vi "3 D Ang Pos for 6 Field-Int.vi"(6 "With Respect To:":enum16{"Referenced", "UnReferenced"}(ring), 7 "LE and RE 2D coils":bool, 8 "Reference index":i32, 9 "3D Convention":T1(ring), 10 "Field Gains":i32[](array[numeric]), 11 "3D Voltage Data":dbl[][](array[numeric]) format="%.2f") -> (3 "3D Position":dbl[][](array[numeric]) format="%.2f")   [LabVIEW 2016]
panel:
  # "Copyright Americo A. Migliaccio (c) 2002 All Rights Reserved by Author"
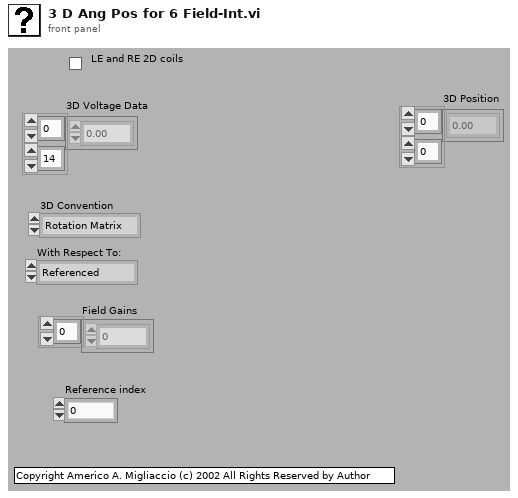
[diagram p1: front panel]
types:
  T1 = enum16{"Rotation Matrix", "Rotation Vectors", "Quaternions", "Fick Angles", "Helmholtz Angles"}
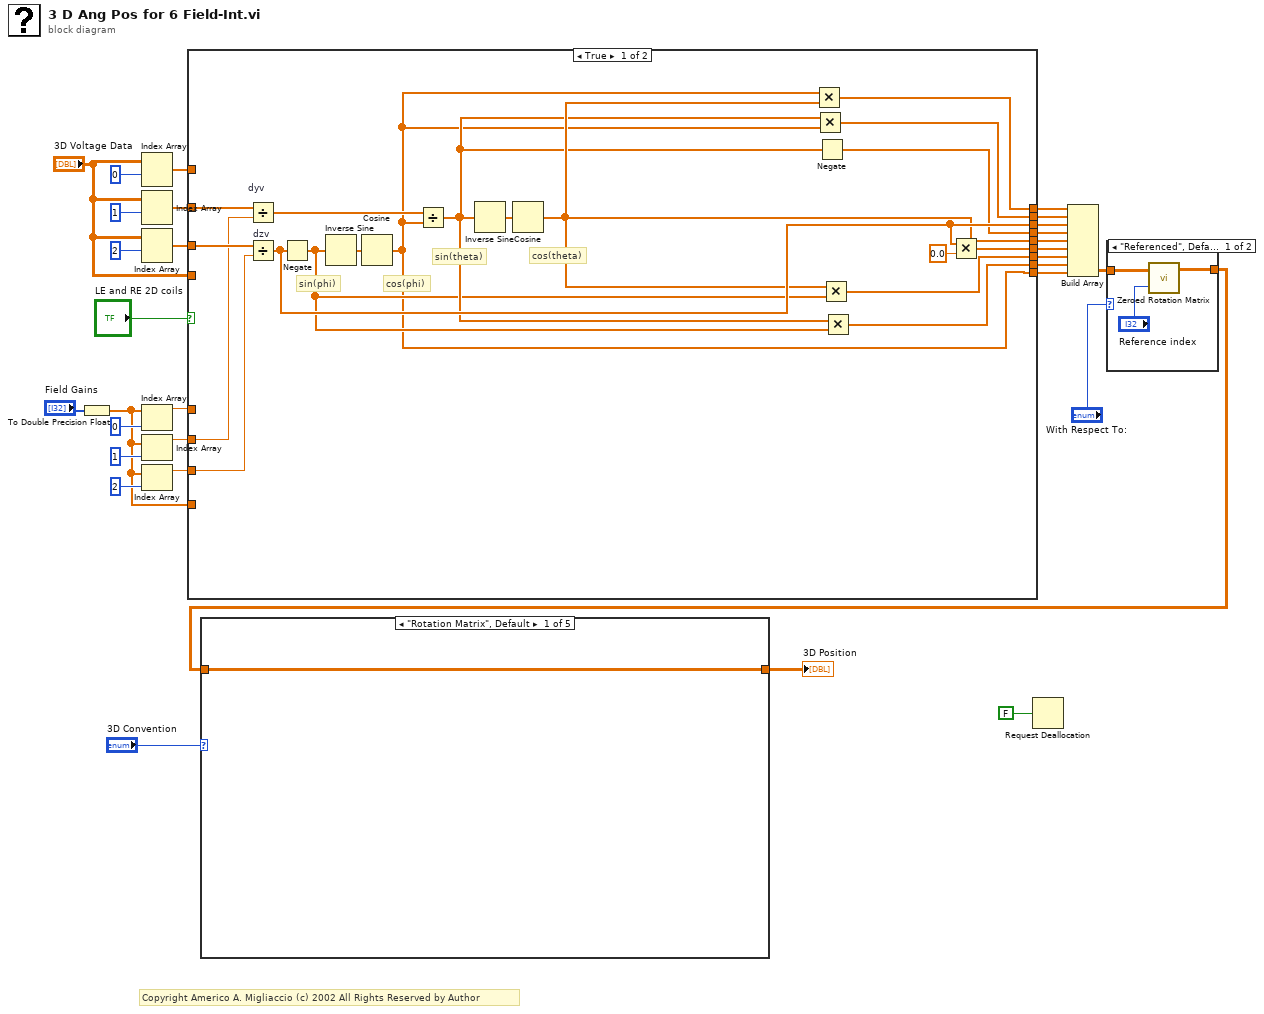
[diagram p0: block diagram]
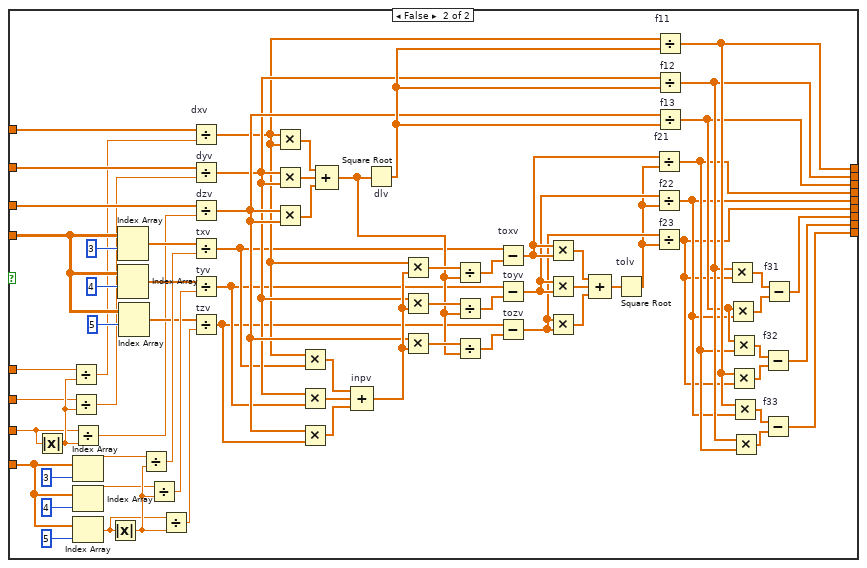
[diagram p2: hidden frame]
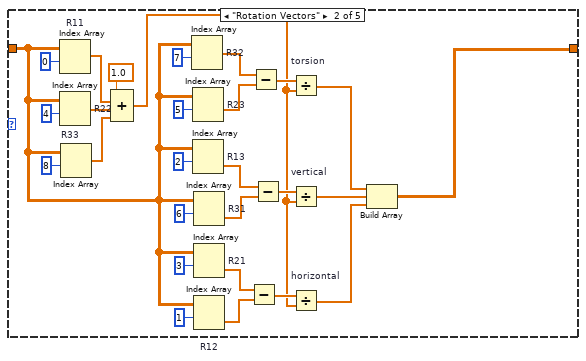
[diagram p4: hidden frame]
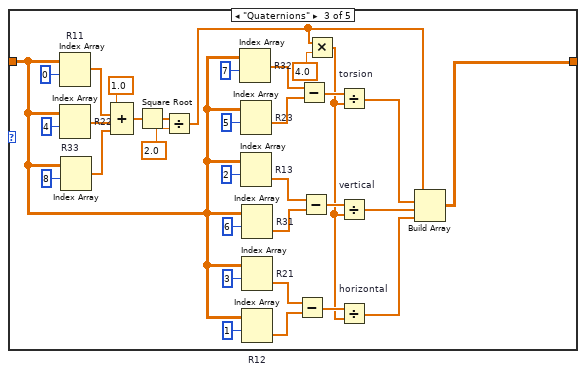
[diagram p5: hidden frame]
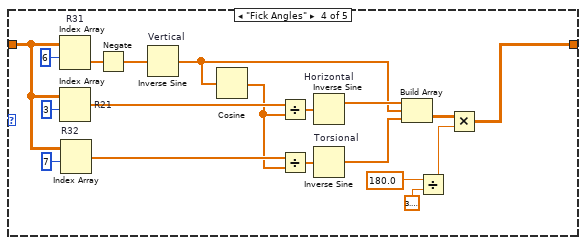
[diagram p6: hidden frame]
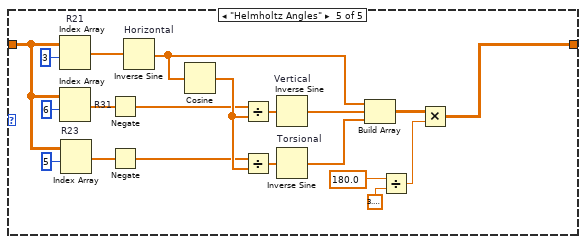
[diagram p7: hidden frame]
diagram:
  # "Copyright Americo A. Migliaccio (c) 2002 All Rights Reserved by Author"
  n1 = To Double Precision Float(number="Field Gains") -> (double precision float=w5:dbl[])
  n2 = Index Array(array="3D Voltage Data", index (row)=0 ("Index (row)")) -> (element=w9:dbl[])  [unwired: 1 in]
  n3 = Index Array(array="3D Voltage Data", index (row)=1 ("Index (row)")) -> (element=w31:dbl[])  [unwired: 1 in]
  n4 = Index Array(array="3D Voltage Data", index (row)=2 ("Index (row)")) -> (element=w30:dbl[])  [unwired: 1 in]
  n5 = Index Array(array=w5, index=0 ("Index")) -> (element=w1:dbl)
  n6 = Index Array(array=w5, index=1 ("Index")) -> (element=w2:dbl)
  n7 = Index Array(array=w5, index=2 ("Index")) -> (element=w3:dbl)
  n8 = case shown="True" "LE and RE 2D coils" {
    tunnel: w31 -> [w50 w122]
    tunnel: w30 -> [w49 w121]
    tunnel: w1 -> [_ w56]
    tunnel: w2 -> [w44 w55]
    tunnel: w3 -> [w43 w54]
    tunnel: [w42 w83] -> w22
    tunnel: [w41 w82] -> w21
    tunnel: [w40 w81] -> w20
    tunnel: [w32 w80] -> w19
    tunnel: [w38 w79] -> w18
    tunnel: [w39 w78] -> w17
    tunnel: [w37 w77] -> w16
    tunnel: [w34 w76] -> w15
    tunnel: [w33 w75] -> w14
    tunnel: w9 -> [_ w74]
    tunnel: "3D Voltage Data" -> [_ w59]
    tunnel: w5 -> [_ w58]
    frame True {
      # "sin(phi)"
      # "cos(phi)"
      # "cos(theta)"
      # "sin(theta)"
      n9 = Divide "dyv"(x=w50, y=w44) -> (x/y=w48:dbl[])
      n10 = Divide "dzv"(x=w49, y=w43) -> (x/y=w40:dbl[])
      n11 = Negate(x=w40) -> (-x=w35:dbl[])
      n12 = Inverse Sine(1:w35) -> (0:w47:dbl[])
      n13 = Cosine(x=w47) -> (cos(x)=w33:dbl[])
      n14 = Divide(x=w48, y=w33) -> (x/y=w36:dbl[])
      n15 = Inverse Sine(1:w36) -> (0:w46:dbl[])
      n16 = Cosine(x=w46) -> (cos(x)=w38:dbl[])
      n17 = Multiply(x=w33, y=w38) -> (x*y=w42:dbl[])
      n18 = Multiply(x=w36, y=w33) -> (x*y=w41:dbl[])
      n19 = Negate(x=w36) -> (-x=w32:dbl[])
      n20 = Multiply(x=w38, y=w35) -> (x*y=w37:dbl[])
      n21 = Multiply(x=w36, y=w35) -> (x*y=w34:dbl[])
      n22 = Multiply(x=w40, y=0.0 ("Index")) -> (x*y=w39:dbl[])
    }
    frame False {
      n23 = Absolute Value(x=w54) -> (abs(x)=w57:dbl)
      n24 = Divide(x=w56, y=w57) -> (x/y=w53:dbl)
      n25 = Divide(x=w55, y=w57) -> (x/y=w52:dbl)
      n26 = Divide(x=w54, y=w57) -> (x/y=w51:dbl)
      n27 = Index Array(array=w58, index=3 ("Index")) -> (element=w117:dbl)
      n28 = Index Array(array=w58, index=4 ("Index")) -> (element=w116:dbl)
      n29 = Index Array(array=w58, index=5 ("Index")) -> (element=w115:dbl)
      n30 = Absolute Value(x=w115) -> (abs(x)=w118:dbl)
      n31 = Index Array(array=w59, index (row)=3 ("Index (row)")) -> (element=w120:dbl[])  [unwired: 1 in]
      n32 = Index Array(array=w59, index (row)=4 ("Index (row)")) -> (element=w119:dbl[])  [unwired: 1 in]
      n33 = Index Array(array=w59, index (row)=5 ("Index (row)")) -> (element=w71:dbl[])  [unwired: 1 in]
      n34 = Divide(x=w117, y=w118) -> (x/y=w114:dbl)
      n35 = Divide(x=w116, y=w118) -> (x/y=w113:dbl)
      n36 = Divide(x=w115, y=w118) -> (x/y=w112:dbl)
      n37 = Divide "dxv"(x=w74, y=w53) -> (x/y=w70:dbl[])
      n38 = Divide "dyv"(x=w122, y=w52) -> (x/y=w72:dbl[])
      n39 = Divide "dzv"(x=w121, y=w51) -> (x/y=w73:dbl[])
      n40 = Divide "txv"(x=w120, y=w114) -> (x/y=w62:dbl[])
      n41 = Divide "tyv"(x=w119, y=w113) -> (x/y=w61:dbl[])
      n42 = Divide "tzv"(x=w71, y=w112) -> (x/y=w60:dbl[])
      n43 = Multiply(x=w70, y=w70) -> (x*y=w105:dbl[])
      n44 = Multiply(x=w72, y=w72) -> (x*y=w104:dbl[])
      n45 = Multiply(x=w73, y=w73) -> (x*y=w103:dbl[])
      n46 = Multiply(x=w70, y=w62) -> (x*y=w102:dbl[])
      n47 = Multiply(x=w72, y=w61) -> (x*y=w101:dbl[])
      n48 = Multiply(x=w73, y=w60) -> (x*y=w100:dbl[])
      n49 = Compound Arithmetic op=ADD ("dlv")(w105, w104, w103) -> (w66:dbl[])
      n50 = Compound Arithmetic op=ADD "inpv"(w102, w101, w100) -> (w99:dbl[])
      n51 = Square Root "dlv"(x=w66) -> (sqrt(x)=w94:dbl[])
      n52 = Multiply(x=w70, y=w99) -> (x*y=w69:dbl[])
      n53 = Multiply(x=w72, y=w99) -> (x*y=w68:dbl[])
      n54 = Multiply(x=w73, y=w99) -> (x*y=w67:dbl[])
      n55 = Divide(x=w69, y=w66) -> (x/y=w65:dbl[])
      n56 = Divide(x=w68, y=w66) -> (x/y=w64:dbl[])
      n57 = Divide(x=w67, y=w66) -> (x/y=w63:dbl[])
      n58 = Subtract "toxv"(x=w62, y=w65) -> (x-y=w93:dbl[])
      n59 = Subtract "toyv"(x=w61, y=w64) -> (x-y=w92:dbl[])
      n60 = Subtract "tozv"(x=w60, y=w63) -> (x-y=w91:dbl[])
      n61 = Multiply(x=w93, y=w93) -> (x*y=w97:dbl[])
      n62 = Multiply(x=w92, y=w92) -> (x*y=w98:dbl[])
      n63 = Multiply(x=w91, y=w91) -> (x*y=w96:dbl[])
      n64 = Compound Arithmetic op=ADD ("dlv")(w97, w98, w96) -> (w95:dbl[])
      n65 = Square Root "tolv"(x=w95) -> (sqrt(x)=w90:dbl[])
      n66 = Divide "f21"(x=w93, y=w90) -> (x/y=w80:dbl[])
      n67 = Divide "f22"(x=w92, y=w90) -> (x/y=w79:dbl[])
      n68 = Divide "f23"(x=w91, y=w90) -> (x/y=w78:dbl[])
      n69 = Divide "f11"(x=w70, y=w94) -> (x/y=w83:dbl[])
      n70 = Divide "f12"(x=w72, y=w94) -> (x/y=w82:dbl[])
      n71 = Divide "f13"(x=w73, y=w94) -> (x/y=w81:dbl[])
      n72 = Multiply(x=w82, y=w78) -> (x*y=w89:dbl[])
      n73 = Multiply(x=w81, y=w79) -> (x*y=w88:dbl[])
      n74 = Multiply(x=w81, y=w80) -> (x*y=w87:dbl[])
      n75 = Multiply(x=w83, y=w78) -> (x*y=w86:dbl[])
      n76 = Multiply(x=w83, y=w79) -> (x*y=w85:dbl[])
      n77 = Multiply(x=w82, y=w80) -> (x*y=w84:dbl[])
      n78 = Subtract "f32"(x=w87, y=w86) -> (x-y=w76:dbl[])
      n79 = Subtract "f33"(x=w85, y=w84) -> (x-y=w75:dbl[])
      n80 = Subtract "f31"(x=w89, y=w88) -> (x-y=w77:dbl[])
    }
  }
  n81 = Request Deallocation(FALSE ("flag")) -> ()
  n82 = Build Array(w22, w21, w20, w19, w18, w17, w16, w15, w14) -> (w13:dbl[][])
  n83 = case shown="\"Referenced\", Default" "With Respect To:" {
    tunnel: w13 -> [w125 w126]
    tunnel: [w123 w126] -> w8
    frame "Referenced", Default {
      n84 = call "Zeroed Rotation Matrix.vi"("Reference index"="Reference index", "Unreferenced Rotation Matrix"=w125) -> ("Referenced Rotation Matrix"=w123:dbl[][])  [unwired: 1 in]
    }
    frame "UnReferenced" {
    }
  }
  n85 = case shown="\"Rotation Matrix\", Default" "3D Convention" {
    tunnel: w8 -> [w127 w142 w175 w204 w224]
    tunnel: [w127 w128 w161 w189 w208] -> w11
    frame "Rotation Matrix", Default {
    }
    frame "Rotation Vectors" {
      n86 = Index Array "R11"(array=w142, index (row)=0 ("Index (row)")) -> (element=w150:dbl[])  [unwired: 1 in]
      n87 = Index Array "R22"(array=w142, index (row)=4 ("Index (row)")) -> (element=w151:dbl[])  [unwired: 1 in]
      n88 = Index Array "R33"(array=w142, index (row)=8 ("Index (row)")) -> (element=w152:dbl[])  [unwired: 1 in]
      n89 = Compound Arithmetic op=ADD(1.0, w150, w151, w152) -> (w132:dbl[])
      n90 = Index Array "R32"(array=w142, index (row)=7 ("Index (row)")) -> (element=w141:dbl[])  [unwired: 1 in]
      n91 = Index Array "R23"(array=w142, index (row)=5 ("Index (row)")) -> (element=w140:dbl[])  [unwired: 1 in]
      n92 = Index Array "R13"(array=w142, index (row)=2 ("Index (row)")) -> (element=w139:dbl[])  [unwired: 1 in]
      n93 = Index Array "R31"(array=w142, index (row)=6 ("Index (row)")) -> (element=w138:dbl[])  [unwired: 1 in]
      n94 = Index Array "R21"(array=w142, index (row)=3 ("Index (row)")) -> (element=w137:dbl[])  [unwired: 1 in]
      n95 = Index Array "R12"(array=w142, index (row)=1 ("Index (row)")) -> (element=w136:dbl[])  [unwired: 1 in]
      n96 = Subtract(x=w137, y=w136) -> (x-y=w133:dbl[])
      n97 = Subtract(x=w141, y=w140) -> (x-y=w135:dbl[])
      n98 = Subtract(x=w139, y=w138) -> (x-y=w134:dbl[])
      n99 = Divide "torsion"(x=w135, y=w132) -> (x/y=w131:dbl[])
      n100 = Divide "vertical"(x=w134, y=w132) -> (x/y=w130:dbl[])
      n101 = Divide "horizontal"(x=w133, y=w132) -> (x/y=w129:dbl[])
      n102 = Build Array(w131, w130, w129) -> (w128:dbl[][])
    }
    frame "Quaternions" {
      n103 = Index Array "R11"(array=w175, index (row)=0 ("Index (row)")) -> (element=w183:dbl[])  [unwired: 1 in]
      n104 = Index Array "R22"(array=w175, index (row)=4 ("Index (row)")) -> (element=w184:dbl[])  [unwired: 1 in]
      n105 = Index Array "R33"(array=w175, index (row)=8 ("Index (row)")) -> (element=w185:dbl[])  [unwired: 1 in]
      n106 = Compound Arithmetic op=ADD(1.0, w183, w184, w185) -> (w165:dbl[])
      n107 = Square Root(x=w165) -> (sqrt(x)=w160:dbl[])
      n108 = Divide(x=w160, y=2.0) -> (x/y=w157:dbl[])
      n109 = Index Array "R32"(array=w175, index (row)=7 ("Index (row)")) -> (element=w174:dbl[])  [unwired: 1 in]
      n110 = Index Array "R23"(array=w175, index (row)=5 ("Index (row)")) -> (element=w173:dbl[])  [unwired: 1 in]
      n111 = Index Array "R13"(array=w175, index (row)=2 ("Index (row)")) -> (element=w172:dbl[])  [unwired: 1 in]
      n112 = Index Array "R31"(array=w175, index (row)=6 ("Index (row)")) -> (element=w171:dbl[])  [unwired: 1 in]
      n113 = Index Array "R21"(array=w175, index (row)=3 ("Index (row)")) -> (element=w170:dbl[])  [unwired: 1 in]
      n114 = Index Array "R12"(array=w175, index (row)=1 ("Index (row)")) -> (element=w169:dbl[])  [unwired: 1 in]
      n115 = Subtract(x=w170, y=w169) -> (x-y=w166:dbl[])
      n116 = Subtract(x=w174, y=w173) -> (x-y=w168:dbl[])
      n117 = Subtract(x=w172, y=w171) -> (x-y=w167:dbl[])
      n118 = Multiply(x=w157, y=4.0) -> (x*y=w156:dbl[])
      n119 = Divide "torsion"(x=w168, y=w156) -> (x/y=w164:dbl[])
      n120 = Divide "vertical"(x=w167, y=w156) -> (x/y=w163:dbl[])
      n121 = Divide "horizontal"(x=w166, y=w156) -> (x/y=w162:dbl[])
      n122 = Build Array(w157, w164, w163, w162) -> (w161:dbl[][])
    }
    frame "Fick Angles" {
      n123 = Index Array "R31"(array=w204, index (row)=6 ("Index (row)")) -> (element=w203:dbl[])  [unwired: 1 in]
      n124 = Index Array "R21"(array=w204, index (row)=3 ("Index (row)")) -> (element=w201:dbl[])  [unwired: 1 in]
      n125 = Index Array "R32"(array=w204, index (row)=7 ("Index (row)")) -> (element=w199:dbl[])  [unwired: 1 in]
      n126 = Negate(x=w203) -> (-x=w202:dbl[])
      n127 = Inverse Sine "Vertical"(1:w202) -> (0:w194:dbl[])
      n128 = Cosine(x=w194) -> (cos(x)=w198:dbl[])
      n129 = Divide(x=w201, y=w198) -> (x/y=w200:dbl[])
      n130 = Divide(x=w199, y=w198) -> (x/y=w197:dbl[])
      n131 = Inverse Sine "Horizontal"(1:w200) -> (0:w196:dbl[])
      n132 = Inverse Sine "Torsional"(1:w197) -> (0:w195:dbl[])
      n133 = Build Array(w196, w194, w195) -> (w193:dbl[][])
      n134 = Divide(x=180.0, y=3.141592653589793) -> (x/y=w190:dbl)
      n135 = Multiply(x=w193, y=w190) -> (x*y=w189:dbl[][])
    }
    frame "Helmholtz Angles" {
      n136 = Index Array "R21"(array=w224, index (row)=3 ("Index (row)")) -> (element=w216:dbl[])  [unwired: 1 in]
      n137 = Index Array "R31"(array=w224, index (row)=6 ("Index (row)")) -> (element=w215:dbl[])  [unwired: 1 in]
      n138 = Index Array "R23"(array=w224, index (row)=5 ("Index (row)")) -> (element=w213:dbl[])  [unwired: 1 in]
      n139 = Negate(x=w215) -> (-x=w214:dbl[])
      n140 = Negate(x=w213) -> (-x=w212:dbl[])
      n141 = Inverse Sine "Horizontal"(1:w216) -> (0:w211:dbl[])
      n142 = Cosine(x=w211) -> (cos(x)=w222:dbl[])
      n143 = Divide(x=w214, y=w222) -> (x/y=w223:dbl[])
      n144 = Divide(x=w212, y=w222) -> (x/y=w221:dbl[])
      n145 = Inverse Sine "Vertical"(1:w223) -> (0:w210:dbl[])
      n146 = Inverse Sine "Torsional"(1:w221) -> (0:w209:dbl[])
      n147 = Build Array(w211, w210, w209) -> (w220:dbl[][])
      n148 = Divide(x=180.0, y=3.141592653589793) -> (x/y=w217:dbl)
      n149 = Multiply(x=w220, y=w217) -> (x*y=w208:dbl[][])
    }
  }
  "3D Position" <- w11
